vi "maintenance_sub.vi"(11 "Instance":i32) -> (1 "SADI State":T1(ring), 2 "FT_OK?":bool, 3 "FT_ERROR_ENUM":T2(ring))   [LabVIEW 2025]
uses:
  LVLib/SADI_FW3.lvlib
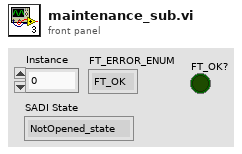
[diagram p1: front panel]
types:
  T1 = enum32{"NotOpened_state", "Opened_state", "Ready_state", "Setup_state", "InitSent_state", "Start_initiated_state", "Run_state", "StopInitiated_state", "Stopped_state"}
  T2 = enum32{"FT_OK", "FT_INVALID_HANDLE", "FT_DEVICE_NOT_FOUND", "FT_DEVICE_NOT_OPENED", "FT_IO_ERROR", "FT_INSUFFICIENT_RESOURCES", "FT_INVALID_PARAMETER", "FT_INVALID_BAUD_RATE", "FT_DEVICE_NOT_OPENED_FOR_ERASE", "FT_DEVICE_NOT_OPENED_FOR_WRITE", "FT_FAILED_TO_WRITE_DEVICE", "FT_EEPROM_READ_FAILED", "FT_EEPROM_WRITE_FAILED", "FT_EEPROM_ERASE_FAILED", "FT_EEPROM_NOT_PRESENT", "FT_EEPROM_NOT_PROGRAMMED", "FT_INVALID_ARGS", "FT_NOT_SUPPORTED", "FT_OTHER_ERROR", "FT_DEVICE_LIST_NOT_READY"}
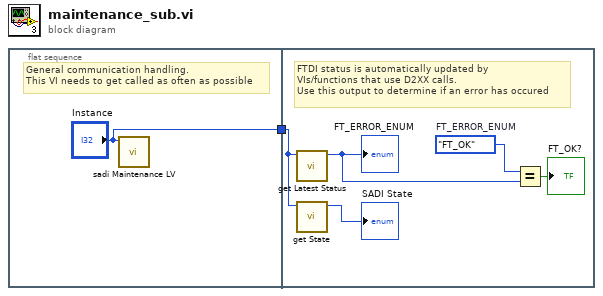
[diagram p0: block diagram]
diagram:
  n1 = flat-sequence {
    tunnel: ["Instance"] -> w1
    tunnel: w1 -> [w3]
    frame #0 {
      # "General communication handling.\nThis VI needs to get called as often as possible"
      n2 = call "sadi Maintenance LV.vi"("instance"="Instance") -> ()  [unwired: 10 in, 1 out]
    }
    frame #1 {
      w6 = T2."FT_OK"  # FT_ERROR_ENUM
      # "FTDI status is automatically updated by\nVIs/functions that use D2XX calls.\nUse this output to determine if an error has occured"
      n3 = call "get Latest Status.vi"("instance"=w3) -> ("function return"=w5:u32)  [unwired: 10 in]
      "FT_ERROR_ENUM" <- w5
      n4 = call "get State.vi"("instance"=w3) -> ("function return"=→"SADI State":u32)  [unwired: 10 in]
      n5 = Equal?(x=w6, y=w5) -> (x = y?=→"FT_OK?":bool)
    }
  }
